vi "WebcamRunning.vi"(10 "NewValue":bool, 11 "Write?":bool) -> (2 "CurrentValue":bool)   [LabVIEW 2013]
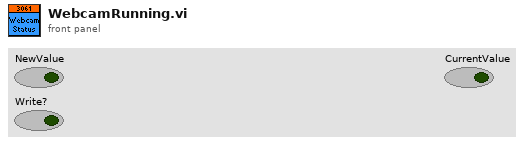
[diagram p1: front panel]
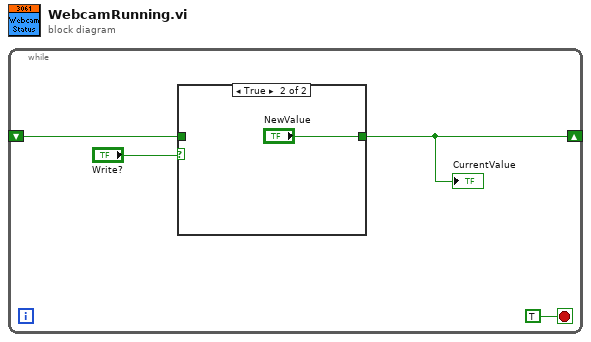
[diagram p0: block diagram]
diagram:
  n1 = while {
    shift-right: [w2] -> _
    shift-left: _ -> [w1]
    stop <- TRUE stop-if-true
    n2 = case shown="True" "Write?" {
      tunnel: [w5 "NewValue"] -> w2
      tunnel: w1 -> [w5 _]
      frame False {
      }
      frame True {
      }
    }
    "CurrentValue" <- w2
  }
